vi "sir_v8.vi"() -> ()   [LabVIEW 2009]
panel:
  out "Numarul in zecimal":dbl
  in  "stop":bool
  in  "Sirul  de caractere care reprezinta un numar in zecimal":string="Extragerea unui subsir din cadrul unui sir de caractere"
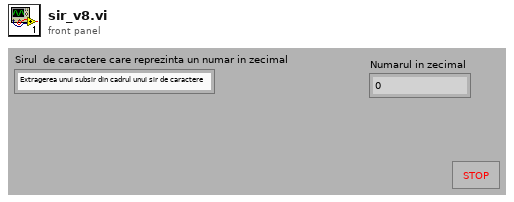
[diagram p1: front panel]
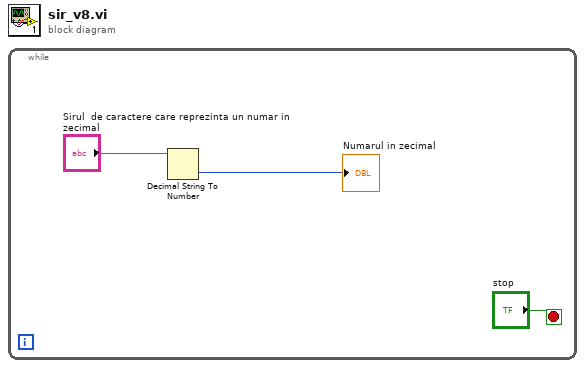
[diagram p0: block diagram]
diagram:
  n1 = while {
    stop <- "stop" stop-if-true
    n2 = Decimal String To Number(string="Sirul  de caractere care reprezinta un numar in zecimal") -> (number=→"Numarul in zecimal":i32)  [unwired: 2 in, 1 out]
  }
